vi "BTESt.vi"(8 "error in (no error)":errorcluster, 10 "Combo Box":string(combo), 11 "VISA resource name":refnum<visa-resource-name>) -> (0 "error out":errorcluster, 3 "VISA resource name out":refnum<visa-resource-name>)   [LabVIEW 2024, in "EFmeter.lvlib"]
uses:
  <instrlib>/EFmeter/EFmeter.lvlib
panel:
  out "Error Message":string
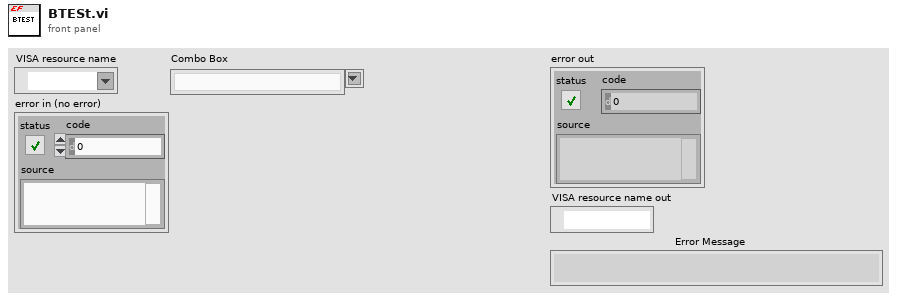
[diagram p1: front panel]
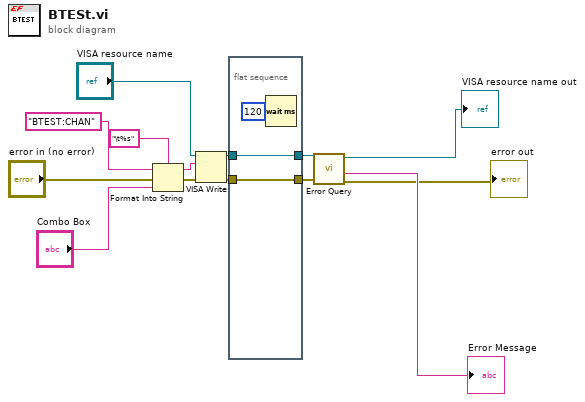
[diagram p0: block diagram]
diagram:
  n1 = Format Into String(format string="\t%s", initial string="BTEST:CHAN", error in="error in (no error)", "Combo Box") -> (resulting string=w8:string, error out=w12:errorcluster)
  n2 = VISA Write(VISA resource name="VISA resource name", write buffer=w8, error in (no error)=w12) -> (VISA resource name out=w7:refnum<visa-resource-name>, error out=w6:errorcluster)  [unwired: 1 out]
  n3 = flat-sequence {
    tunnel: w7 -> [w17]
    tunnel: [w17] -> w4
    tunnel: [w16] -> w5
    tunnel: w6 -> [w16]
    frame #0 {
      n4 = Wait (ms)(milliseconds to wait=u32 120) -> ()  [unwired: 1 out]
    }
  }
  n5 = call <instrlib>:"Error Query.vi"("error in (no error)"=w5, "VISA resource name"=w4) -> ("error out"=→"error out":errorcluster, "Error Message"=→"Error Message":string, "VISA resource name out"=→"VISA resource name out":refnum<visa-resource-name>)  [unwired: 6 in, 1 out]
